vi "AR-Select-Single-DO.vi"(6 "error in (no error)":errorcluster, 7 "Action":T1, 10 "DO":bool, 11 "index":i32) -> (2 "error out":errorcluster, 3 "DO Data":bool[](array[boolean]))   [LabVIEW 2021]
uses:
  Controls/AR-DO-Action.ctl
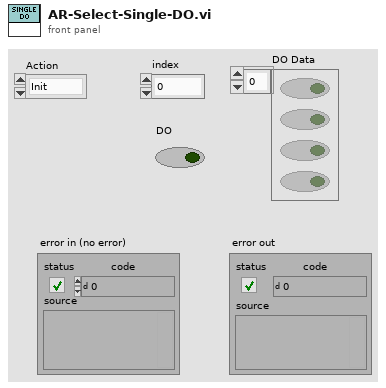
[diagram p1: front panel]
types:
  T1 = typedef "AR-DO-Action.ctl" = enum16{"Init", "Update", "Keep DO3", "Idle"}
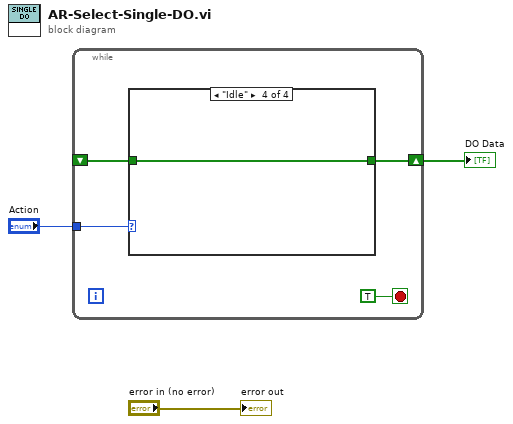
[diagram p0: block diagram]
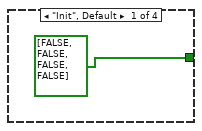
[diagram p2: hidden frame]
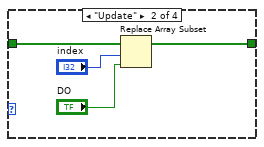
[diagram p3: hidden frame]
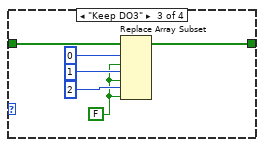
[diagram p4: hidden frame]
diagram:
  n1 = while {
    tunnel: "Action" -> [w6]
    shift-right: [w5] -> w2
    shift-left: _ -> [w4]
    stop <- TRUE stop-if-true
    n2 = case shown="\"Idle\"" w6 {
      tunnel: [bool[] [FALSE, FALSE, FALSE, FALSE] ("Data") w9 w17 w19] -> w5
      tunnel: w4 -> [_ w11 w18 w19]
      frame "Init", Default {
      }
      frame "Update" {
        n3 = Replace Array Subset(array=w11, new element="DO", index="index") -> (w9:bool[])
      }
      frame "Keep DO3" {
        w13 = FALSE
        n4 = Replace Array Subset(array=w18, new element #1=w13, index #1=0 ("index"), new element #2=w13, index #2=1 ("index"), new element #3=w13, index #3=2 ("index")) -> (w17:bool[])
      }
      frame "Idle" {
      }
    }
  }
  "DO Data" <- w2
  "error out" <- "error in (no error)"
